vi "get Last Error.vi"(8 "error in (no error)":errorcluster, 11 "error_code":u16) -> (0 "error out":errorcluster, 2 "function return":bool, 3 "error_code out":u16)   [LabVIEW 2015, in "XGL_DPP.lvlib"]
doc: "EXTERN DECLSPEC bool CALL_CONV getLastError(unsigned short int& error_code);"
uses:
  XGL_DPP.lvlib
  XGL_DPP.dll
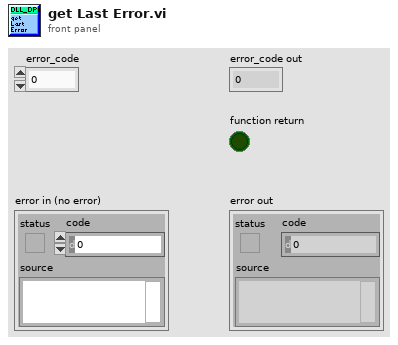
[diagram p1: front panel]
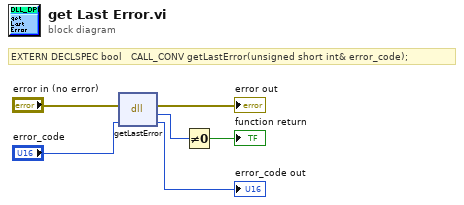
[diagram p0: block diagram]
diagram:
  # "EXTERN DECLSPEC bool   CALL_CONV getLastError(unsigned short int& error_code);"
  n1 = dll-call lib="D:/Users/XRF/Desktop/Dante_acquire4/libs/Dante/XGL_DPP.*" fn="getLastError"(error in="error in (no error)", "error_code"="error_code") -> (error out=→"error out":errorcluster, "return type"=w5:u8, "error_code"=→"error_code out":u16)  [unwired: 2 in, 1 out]
  n2 = Not Equal To 0?(x=w5) -> (x != 0?=→"function return":bool)
